vi "Vision Processing.vi"(4 "error in (no error)":errorcluster, 6 "CameraDevRef":T1) -> ()   [LabVIEW 2011]
uses:
  <vilib>/Rock Robotics/WPI/Camera/WPI_CameraDevRef.ctl
  Robot Global Data.vi
  <vilib>/vision/NI_Vision_Development_Module.lvlib
panel:
  in  "Run Calculations":bool
  in  "Manual Overide":bool
  out "Raw Turret":dbl
  out "Target X Coord":dbl
  out "Target Distance":dbl
  out "Target Y Coord":dbl
  out "Distance Array":dbl[](array[numeric])
  in  "Scaler":dbl=0.85
  in  "Lower Speed Limit":dbl=0.05
  out "Number of Rectangles Visible":dbl
  out "Y Position Array":dbl[](array[numeric])
  out "X Position Array":dbl[](array[numeric])
  in  "View":bool
  out "Target Info":T2(array[cluster])
  in  "Area Size Limit":i32=444
  in  "Particle Count Limit":i32=8
  in  "Score Limits":T3={"Rect Coverage"=76.0, "Aspect Ratio"=40.0, "X Edge Strength"=40.0, "Y Edge Strength"=60.0}
  in  "Processing":enum32{"Color", "Intensity", "Intensity Open"}(tab)=enum."Intensity Open"
  in  "Luminance":i32=255
  in  "Saturation":i32=255
  in  "Hue":i32(knob)=65 scale=0.0..255.0
  in  "Margins":cluster{"Hue":i32, "Sat":i32, "Lum":i32}={"Hue"=20, "Sat"=27, "Lum"=30} {"Sat" scale=0.0..40.0; "Lum" scale=0.0..40.0; "Hue" scale=0.0..40.0}
  in  "Range":cluster{"Lower value":sgl, "Upper value":sgl}={"Lower value"=150.0, "Upper value"=255.0} {"Lower value" scale=0.0..255.0; "Upper value" scale=0.0..255.0}
  in  "Range":cluster{"Lower value":sgl, "Upper value":sgl}={"Lower value"=123.804344, "Upper value"=255.0} {"Lower value" scale=0.0..255.0; "Upper value" scale=0.0..255.0}
  in  "View":bool
  out "Processed Image":T4(plugin-control)
  out "Original Image":T4(plugin-control)
  # "Instructions:\nProcessing the reflective tape that is illuminated by a ring light can be based\non color or light intensity.\nParticles within the image are scored by rectangle coverage, aspect ratio, and\nfor being hollow with a bold edge. A particle is considered a target if all scores\nare above the score limits. Particles can be annotated -- surrounded by\na rectangle and scores drawn to the left .\nTo control the number of particles being scored, use the count limit and the size\nlimit."
  # "To debug, Enable using the View button.\nFor color processing, you can click in the image to select the color for processing."
  # "Enable by clicking the View button.\nGreen scores are above the limit, orange are below. Inner/outer rect\nindicates all passed."
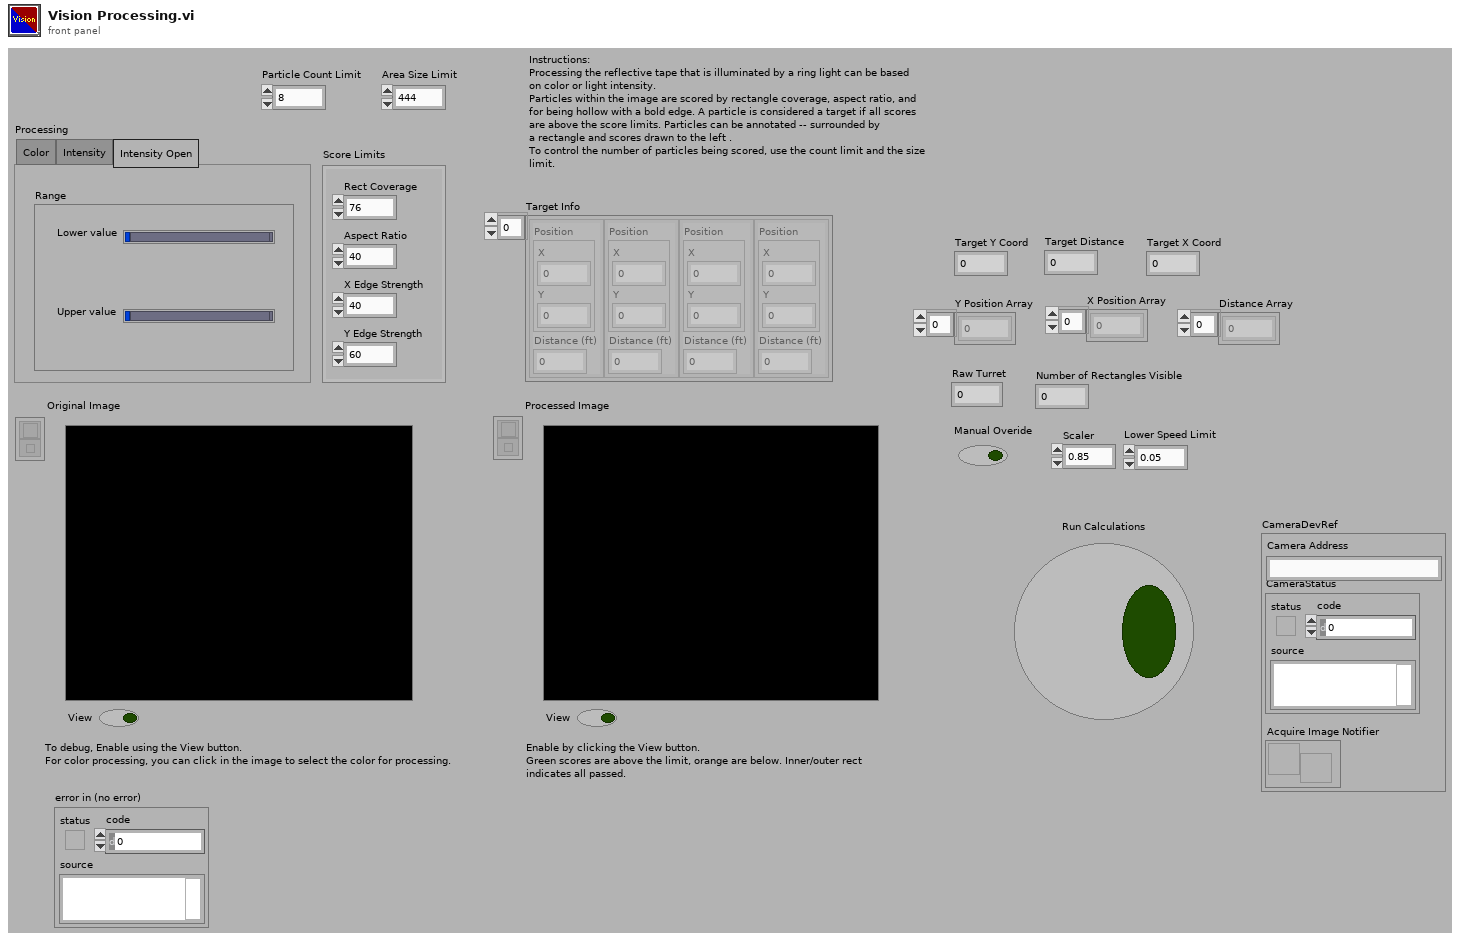
[diagram p1: front panel]
types:
  T1 = typedef "WPI_CameraDevRef.ctl" = cluster{"Camera Address":string, "CameraStatus":errorcluster, "Acquire Image Notifier":refnum<notifier>}
  T2 = cluster{"Position":cluster{"X":dbl, "Y":dbl}, "Distance (ft)":dbl}[]
  T3 = cluster{"Rect Coverage":dbl, "Aspect Ratio":dbl, "X Edge Strength":dbl, "Y Edge Strength":dbl}
  T4 = typedef "IMAQ Image.ctl" = refnum<image>
  T5 = typedef "Image Type" = u32
  T6 = enum32{"AutoM", "Close", "Dilate", "Erode", "Gradient", "Gradient out", "Gradient in", "Hit miss", "Open", "PClose", "POpen", "Thick", "Thin"}
  T7 = typedef "WPI_CameraImageSize.ctl" = enum16{"640x480", "320x240", "160x120"}
  T8 = cluster{"fps":i32, "compression":i32, "Image Size":T7}
  T9 = cluster{cluster{"Left":dbl, "Top":dbl, "Right":dbl, "Bottom":dbl}, dbl[]}[]
  T10 = cluster{"Left":dbl, "Top":dbl, "Right":dbl, "Bottom":dbl}
  T11 = cluster{"Target Center (-1 to 1)":cluster{"X":dbl, "Y":dbl}, "Distance (ft)":dbl}
  T12 = cluster{"Target Center (-1 to 1)":cluster{"X":dbl, "Y":dbl}, "Distance (ft)":dbl}[]
  T13 = cluster{"Axis 1":dbl, "Axis 2":dbl, "Axis 3":dbl, "Axis 4":dbl, "Axis 5":dbl, "Axis 6":dbl, "Button 1":bool, "Button 2":bool, "Button 3":bool, "Button 4":bool, "Button 5":bool, "Button 6":bool, "Button 7":bool, "Button 8":bool, "Button 9":bool, "Button 10":bool, "Button 11":bool, "Button 12":bool}
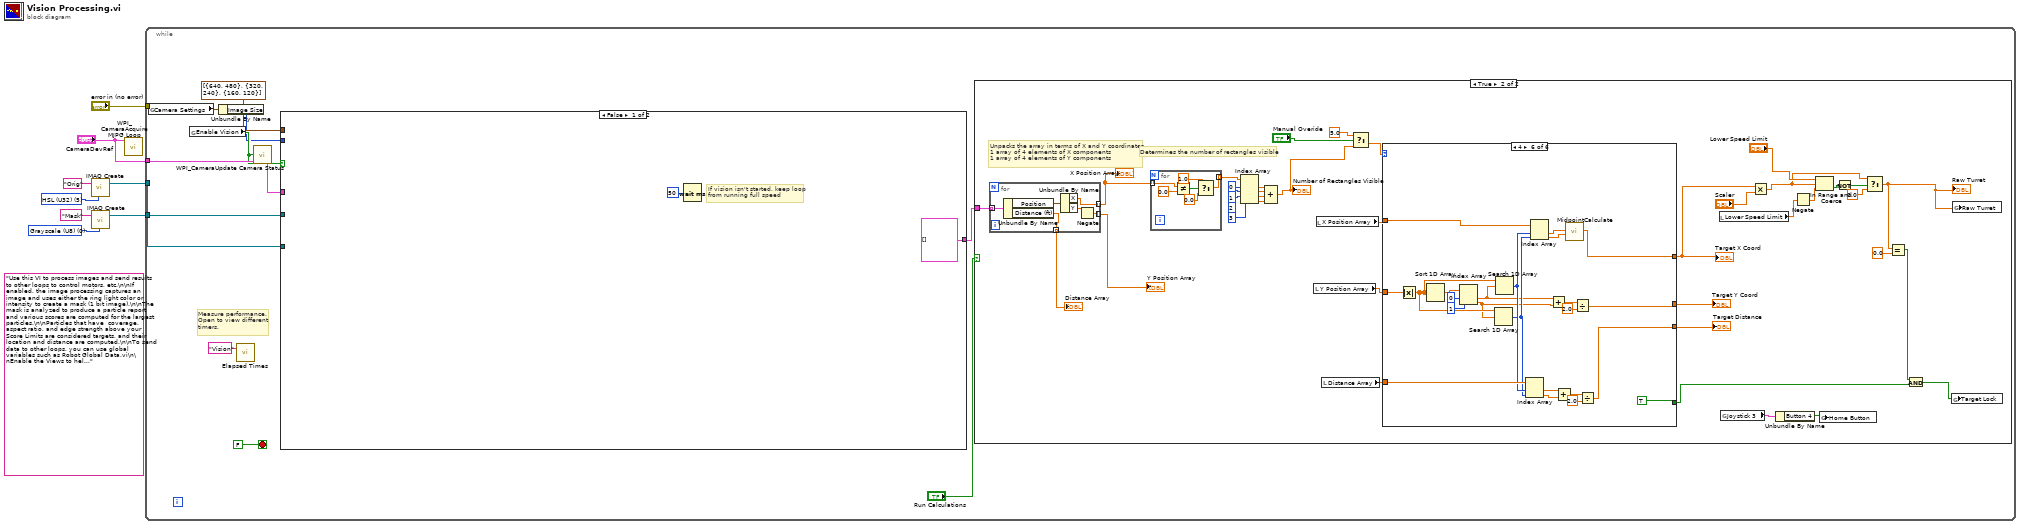
[diagram p0: block diagram]
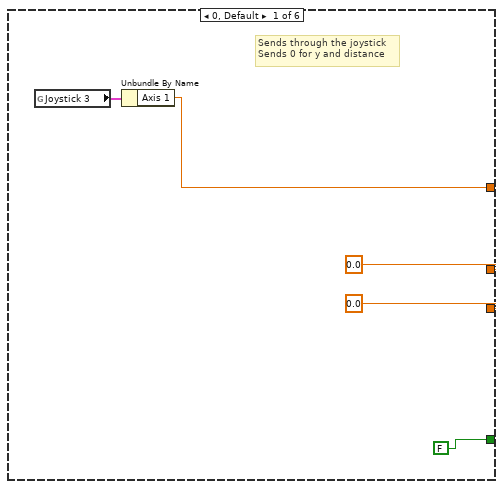
[diagram p3: hidden frame]
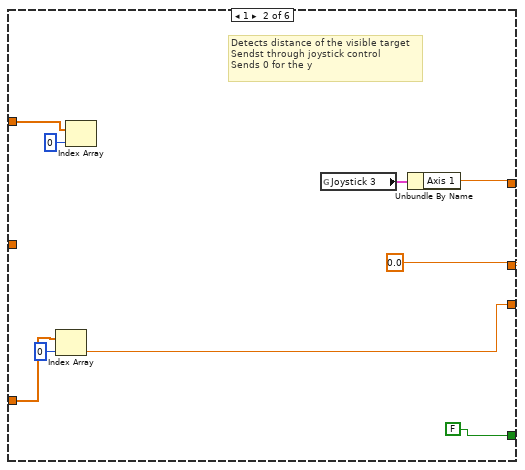
[diagram p4: hidden frame]
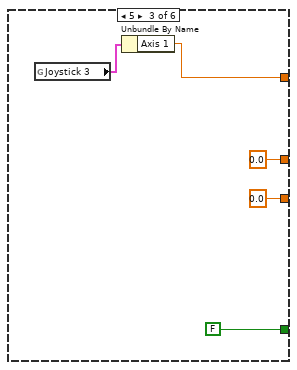
[diagram p5: hidden frame]
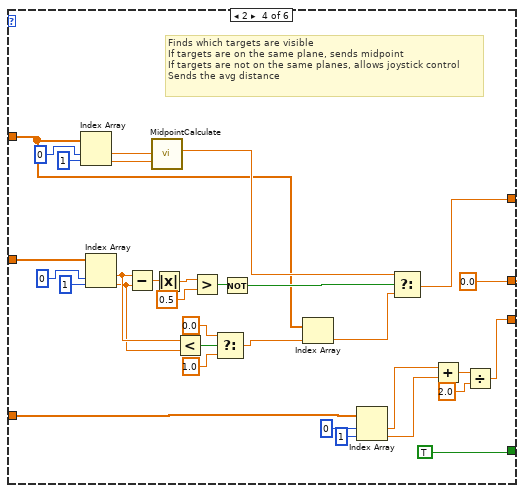
[diagram p6: hidden frame]
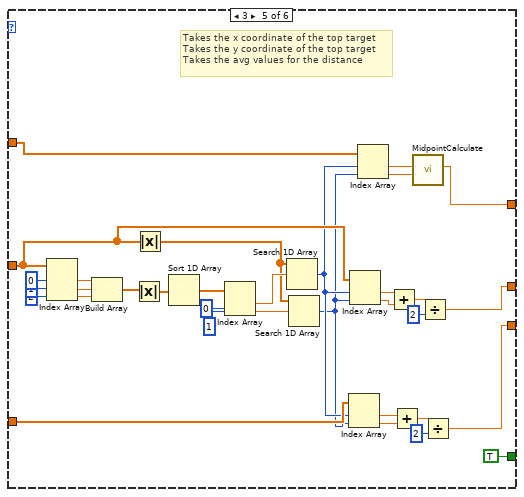
[diagram p7: hidden frame]
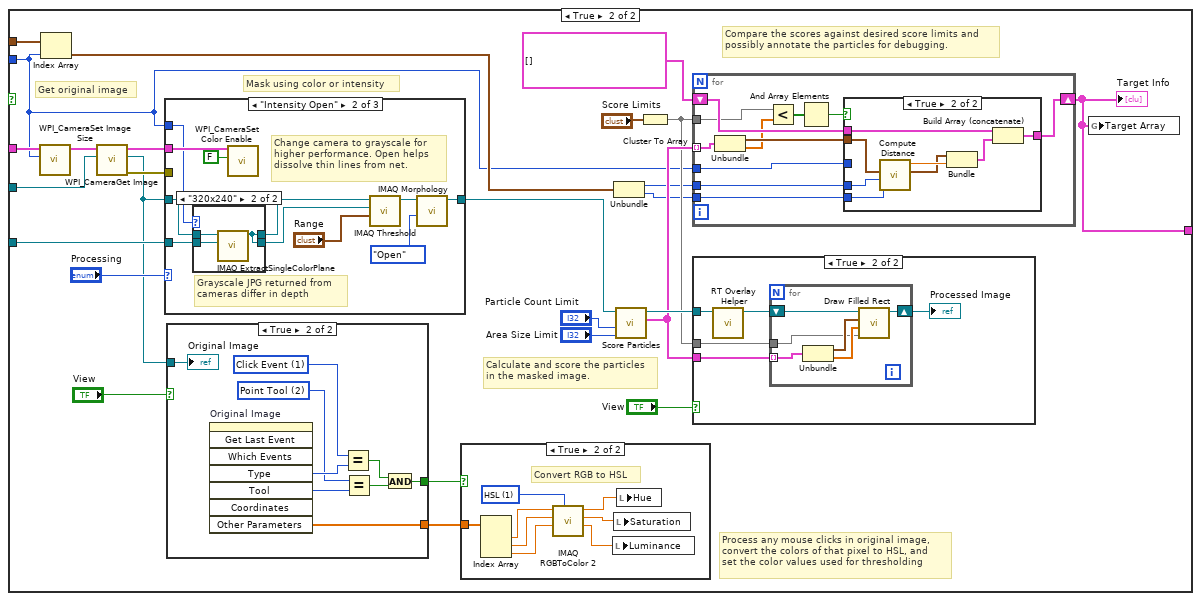
[diagram p8: hidden frame]
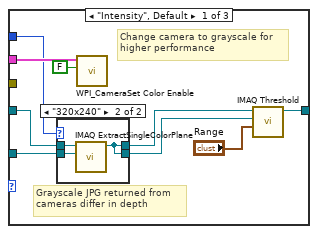
[diagram p10: hidden frame]
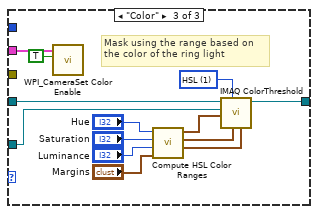
[diagram p13: hidden frame]
diagram:
  w3 = T5 0 items=["Grayscale (U8)", "Grayscale (I16)", "Grayscale (SGL)", "Complex (CSG)", "RGB (U32)", "HSL (U32)", "RGB (U64)", "Grayscale (U16)"] ("Image Type")
  (unwired) "Use this VI to process images and send results to other loops to control motors, etc.\n\nIf enabled, the image processing captures an image and uses either the ring light color or intensity to create a mask (1 bit image).\n\nThe mask is analyzed to produce a particle report and various scores are computed for the largest particles.\n\nParticles that have  coverage, aspect ratio, and edge strength above your Score Limits are considered targets, and their location and distance are computed.\n\nTo send data to other loops, you can use global variables such as Robot Global Data.vi\n\nEnable the Views to help debug color settings. Disable the View to speed up processing."
  w7 = T5 5 items=["Grayscale (U8)", "Grayscale (I16)", "Grayscale (SGL)", "Complex (CSG)", "RGB (U32)", "HSL (U32)", "RGB (U64)", "Grayscale (U16)"] ("Image Type")
  n1 = call "IMAQ Create"("Image Name"="Orig", "Image Type"=w7) -> ("New Image"=w6:T4)  [unwired: 2 in, 2 out]
  n2 = call "IMAQ Create"("Image Name"="Mask", "Image Type"=w3) -> ("New Image"=w1:T4)  [unwired: 2 in, 2 out]
  n3 = call <vilib>:"WPI_CameraAcquire MJPG Loop.vi"("CameraDevRef"="CameraDevRef") -> ()  [unwired: 11 in]
  n4 = while {
    tunnel: w6 -> [w19]
    tunnel: "CameraDevRef" -> [w18]
    tunnel: "error in (no error)" -> [_]
    tunnel: w1 -> [w14]
    stop <- FALSE stop-if-true
    # "Measure performance.\nOpen to view different\ntimers."
    n5 = global read "Robot Global Data.vi" "Camera Settings"() -> (w12:T8)
    n6 = global read "Robot Global Data.vi" "Enable Vision"() -> (w16:bool)
    n7 = Unbundle By Name(w12) -> ("Image Size"=w11:T7)
    n8 = call "Elapsed Times.vi"("Call Name"="Vision") -> ()  [unwired: 2 in, 1 out]
    n9 = call <vilib>:"WPI_CameraUpdate Camera Status.vi"("CameraDevRef In"=w18, "Enable Vision"=w16) -> ("CameraDevRef Out"=w17:T1)  [unwired: 3 in]
    n10 = case shown="False" w16 {
      tunnel: w19 -> [_ w196]
      tunnel: w17 -> [_ w192]
      tunnel: w14 -> [_ w183]
      tunnel: cluster{i32, i32}[] [{640, 480}, {320, 240}, {160, 120}] -> [_ w187]
      tunnel: w11 -> [_ w180]
      tunnel: [T2 [] w181] -> w10
      frame False {
        # "If vision isn't started, keep loop\nfrom running full speed"
        n11 = Wait (ms)(milliseconds to wait=u32 50) -> ()  [unwired: 1 out]
      }
      frame True {
        # "Compare the scores against desired score limits and\npossibly annotate the particles for debugging."
        # "Process any mouse clicks in original image,\nconvert the colors of that pixel to HSL, and\nset the color values used for thresholding"
        # "Calculate and score the particles\nin the masked image."
        # "Mask using color or intensity"
        # "Get original image"
        n12 = call <vilib>:"WPI_CameraSet Image Size.vi"("Image Size"=w180, "CameraDevRef"=w192) -> ("CameraDevRef Out"=w193:T1)  [unwired: 8 in, 1 out]
        n13 = Index Array(array=w187, index=w180) -> (element=w184:cluster{i32, i32})
        n14 = call <vilib>:"WPI_CameraGet Image.vi"("Image"=w196, "CameraDevRef"=w193) -> ("error out"=w194:errorcluster, "Image Out"=w182:T4, "CameraDevRef Out"=w195:T1)  [unwired: 7 in]
        n15 = case shown="\"Intensity Open\"" "Processing" {
          tunnel: w182 -> [w218 w230 w256]
          tunnel: [w221 w235 w255] -> w190
          tunnel: w195 -> [w219 w233 w246]
          tunnel: w194 -> [_ _ _]
          tunnel: w183 -> [w217 w231 w244]
          tunnel: w180 -> [w216 w232 _]
          frame "Intensity", Default {
            # "Grayscale JPG returned from\ncameras differ in depth"
            # "Change camera to grayscale for\nhigher performance"
            n16 = case shown="\"320x240\"" w216 {
              tunnel: w218 -> [w224 w227]
              tunnel: w217 -> [w223 w226]
              tunnel: [w224 w225] -> w215
              tunnel: [w223 w225] -> w214
              frame "640x480", Default {
              }
              frame "320x240" {
                n17 = call "IMAQ ExtractSingleColorPlane"("Image Dst"=w226, "Image Src"=w227) -> ("Image Dst Out"=w225:T4)  [unwired: 8 in, 1 out]
              }
            }
            n18 = call <vilib>:"WPI_CameraSet Color Enable.vi"("Color Enabled"=FALSE, "CameraDevRef"=w219) -> ()  [unwired: 8 in, 2 out]
            n19 = call "IMAQ Threshold"("Range"="Range", "Image Dst"=w214, "Image Src"=w215) -> ("Image Dst Out"=w221:T4)  [unwired: 3 in, 5 out]
          }
          frame "Intensity Open" {
            # "Grayscale JPG returned from\ncameras differ in depth"
            # "Change camera to grayscale for\nhigher performance. Open helps\ndissolve thin lines from net."
            n20 = case shown="\"320x240\"" w232 {
              tunnel: w230 -> [w240 w243]
              tunnel: w231 -> [w239 w242]
              tunnel: [w240 w241] -> w229
              tunnel: [w239 w241] -> w228
              frame "640x480", Default {
              }
              frame "320x240" {
                n21 = call "IMAQ ExtractSingleColorPlane"("Image Dst"=w242, "Image Src"=w243) -> ("Image Dst Out"=w241:T4)  [unwired: 8 in, 1 out]
              }
            }
            n22 = call <vilib>:"WPI_CameraSet Color Enable.vi"("Color Enabled"=FALSE, "CameraDevRef"=w233) -> ()  [unwired: 8 in, 2 out]
            n23 = call "IMAQ Threshold"("Range"="Range", "Image Dst"=w228, "Image Src"=w229) -> ("Image Dst Out"=w236:T4)  [unwired: 3 in, 5 out]
            n24 = call "IMAQ Morphology"("Operation"=T6."Open", "Image Src"=w236) -> ("Image Dst Out"=w235:T4)  [unwired: 8 in, 1 out]
          }
          frame "Color" {
            w254 = u16 1 items=["RGB", "HSL", "HSV", "HSI"] ("Color Mode")
            # "Mask using the range based on\nthe color of the ring light"
            n25 = call <vilib>:"WPI_CameraSet Color Enable.vi"("Color Enabled"=TRUE, "CameraDevRef"=w246) -> ()  [unwired: 8 in, 2 out]
            n26 = call "Compute HSL Color Ranges.vi"("Margins"="Margins", "Luminance"="Luminance", "Saturation"="Saturation", "Hue"="Hue") -> ("Lum Range"=w251:cluster{i32, i32}, "Sat Range"=w252:cluster{i32, i32}, "Hue Range"=w253:cluster{i32, i32})  [unwired: 5 in]
            n27 = call "IMAQ ColorThreshold"("Blue or Luma or Val or Inten Range"=w251, "Green or Sat Range"=w252, "Color Mode"=w254, "Red or Hue Range"=w253, "Image Dst"=w244, "Image Src"=w256) -> ("Image Dst Out"=w255:T4)  [unwired: 4 in, 1 out]
          }
        }
        n28 = case shown="True" "View" {
          tunnel: w182 -> [_ w276]
          tunnel: [_ w271] -> w189
          tunnel: [_ w268] -> w188
          frame False {
          }
          frame True {
            w269 = 2 items=["None", "Selection Tool", "Point Tool", "Line Tool", "Rectangle Tool", "Oval Tool", "Polygon Tool", "ClosedFreehandTool", "Annulus Tool", "Rotated Rectangle Tool", "Zoom Tool", "Pan Tool", "Polyline Tool", "Freehand Tool"] ("Tool")
            w270 = 1 items=["No Event"=0, "Click Event"=1, "Draw Event"=2, "Size Event"=4, "Scroll Event"=5, "Double Click Event"=8] ("Type")
            n29 = invoke on="Original Image" class="ImageControl" method="Get Last Event"() -> ("Type"=w272:i32, "Tool"=w275:i32, "Other Parameters"=w268:sgl[])  [unwired: 8 in, 5 out]
            n30 = Equal?(x=w270, y=w272) -> (x = y?=w273:bool)
            n31 = Equal?(x=w269, y=w275) -> (x = y?=w274:bool)
            n32 = And(x=w273, y=w274) -> (x .and. y?=w271:bool)
            "Original Image" <- w276
          }
        }
        n33 = case shown="True" w189 {
          tunnel: w188 -> [_ w213]
          frame False {
          }
          frame True {
            w212 = u16 1 items=["RGB", "HSL", "HSV", "HSI", "CIE L*a*b*", "CIE XYZ"] ("Color Mode")
            # "Convert RGB to HSL"
            n34 = Index Array(array=w213) -> (element #1=w211:sgl, element #2=w209:sgl, element #3=w207:sgl)  [unwired: 3 in]
            n35 = call "IMAQ RGBToColor 2"("Color Mode"=w212, "Blue value"=w207, "Green value"=w209, "Red value"=w211) -> ("Blue or Luma or Val or Inten or Z or b*value"=w206:dbl, "Green or Sat or Y or a* value"=w208:dbl, "Red or Hue or X or L* value"=w210:dbl)  [unwired: 4 in, 1 out]
            n36 = local write "Luminance"(w206) -> ()
            n37 = local write "Saturation"(w208) -> ()
            n38 = local write "Hue"(w210) -> ()
          }
        }
        n39 = Unbundle(w184) -> (w186:i32, w185:i32)
        n40 = call "Score Particles.vi"("Area Size Limit"="Area Size Limit", "Particle Count Limit"="Particle Count Limit", "Image Refnum in"=w190) -> ("Scored Particle Info"=w201:T9, "Image Refnum out"=w204:T4)  [unwired: 7 in]
        n41 = Cluster To Array(cluster="Score Limits") -> (array=w199:dbl[])
        n42 = for {
          shift-right: [w286] -> w181
          shift-left: T2 [] -> [w287]
          tunnel: w186 -> [w285]
          tunnel: w201 -> [w283] mode=indexing
          tunnel: w199 -> [w278]
          tunnel: w180 -> [w282]
          tunnel: w185 -> [w277]
          n43 = Unbundle(w283) -> (w284:T10, w279:dbl[])
          n44 = Less?(x=w278, y=w279) -> (x < y?=w281:bool[])
          n45 = And Array Elements(Boolean array=w281) -> (logical AND=w280:bool)
          n46 = case shown="True" w280 {
            tunnel: w287 -> [w288 w296]
            tunnel: [w288 w295] -> w286
            tunnel: w284 -> [_ w291]
            tunnel: w285 -> [_ w293]
            tunnel: w282 -> [_ _]
            tunnel: w277 -> [_ w290]
            frame False {
            }
            frame True {
              n47 = call "Compute Distance.vi"("Y Image Resolution"=w290, "X Image Resolution"=w293, "Bounding Box"=w291) -> ("Target Center (-1 to 1)"=w289:cluster{"X":dbl, "Y":dbl}, "Distance (ft)"=w292:dbl)  [unwired: 7 in]
              n48 = Bundle("Target Center (-1 to 1)"=w289, "Distance (ft)"=w292) -> (w294:T11)  [unwired: 1 in]
              n49 = Build Array (concatenate)(w296, w294) -> (w295:T12)
            }
          }
        }
        "Target Info" <- w181
        n50 = case shown="True" "View" {
          tunnel: w204 -> [_ w258]
          tunnel: w201 -> [_ w260]
          tunnel: w199 -> [_ w259]
          frame False {
          }
          frame True {
            n51 = call "RT Overlay Helper.vi"("Refnum in"=w258) -> ("Refnum out"=w261:T4)  [unwired: 10 in]
            n52 = for {
              shift-right: [w266] -> w257
              shift-left: w261 -> [w267]
              tunnel: w260 -> [w263] mode=indexing
              tunnel: w259 -> [w262]
              n53 = Unbundle(w263) -> (w264:T10, w265:dbl[])
              n54 = call "Draw Filled Rect.vi"("Limits"=w262, "Scores"=w265, "Bounding Box"=w264, "image in"=w267) -> ("image out"=w266:T4)  [unwired: 7 in]
            }
            "Processed Image" <- w257
          }
        }
        n55 = global write "Robot Global Data.vi" "Target Array"(w181) -> ()
      }
    }
    n56 = case shown="True" "Run Calculations" {
      tunnel: w10 -> [_ w29]
      frame False {
      }
      frame True {
        # "Determines the number of rectangles visible"
        # "Unpacks the array in terms of X and Y coordinates\n1 array of 4 elements of X components\n1 array of 4 elements of Y components"
        n57 = for {
          tunnel: [w175] -> w30 mode=indexing
          tunnel: [w176] -> w40 mode=indexing
          tunnel: w29 -> [w173] mode=indexing
          tunnel: [w172] -> w49 mode=indexing
          n58 = Unbundle By Name(w173) -> ("Position"=w177:cluster{"X":dbl, "Y":dbl}, "Distance (ft)"=w172:dbl)
          n59 = Unbundle By Name(w177) -> ("X"=w176:dbl, "Y"=w174:dbl)
          n60 = Negate(x=w174) -> (-x=w175:dbl)
        }
        "X Position Array" <- w40
        "Y Position Array" <- w30
        "Distance Array" <- w49
        n61 = for {
          tunnel: w40 -> [w63] mode=indexing
          tunnel: [w59] -> w39 mode=indexing
          n62 = Not Equal?(x=w63, y=0.0) -> (x != y?=w62:bool)
          n63 = Select(t=1.0, s=w62, f=0.0) -> (s? t:f=w59:dbl)
        }
        n64 = Index Array(array=w39, index #1=0 ("index"), index #2=1 ("index"), index #3=2 ("index"), index #4=3 ("index")) -> (element #1=w37:dbl, element #2=w38:dbl, element #3=w36:dbl, element #4=w35:dbl)
        n65 = Compound Arithmetic op=ADD(w37, w38, w36, w35) -> (w28:dbl)
        "Number of Rectangles Visible" <- w28
        n66 = local read "Y Position Array"() -> (w53:dbl[])
        n67 = local read "X Position Array"() -> (w41:dbl[])
        n68 = local read "Distance Array"() -> (w54:dbl[])
        n69 = Select(t=5.0, s="Manual Overide", f=w28) -> (s? t:f=w57:dbl)
        n70 = case shown="4" w57 {
          tunnel: w41 -> [_ w73 _ w86 w132 w165]
          tunnel: [w68 w71 w82 w104 w129 w155] -> w52
          tunnel: [0.0 ("X") 0.0 ("X") 0.0 ("X") 0.0 ("X") w133 w154] -> w50
          tunnel: [0.0 ("X") w76 0.0 ("X") w97 w117 w149] -> w51
          tunnel: w53 -> [_ _ _ w113 w125 w170]
          tunnel: w54 -> [_ w78 _ w96 w120 w164]
          tunnel: [FALSE FALSE FALSE TRUE TRUE TRUE] -> w25
          frame 0, Default {
            # "Sends through the joystick\nSends 0 for y and distance"
            n71 = global read "Robot Global Data.vi" "Joystick 3"() -> (w69:T13)
            n72 = Unbundle By Name(w69) -> ("Axis 1"=w68:dbl)
          }
          frame 1 {
            # "Detects distance of the visible target\nSendst through joystick control\nSends 0 for the y"
            n73 = Index Array(array=w78, index=0) -> (element=w76:dbl)
            n74 = Index Array(array=w73, index=0) -> ()  [unwired: 1 out]
            n75 = global read "Robot Global Data.vi" "Joystick 3"() -> (w72:T13)
            n76 = Unbundle By Name(w72) -> ("Axis 1"=w71:dbl)
          }
          frame 5 {
            n77 = global read "Robot Global Data.vi" "Joystick 3"() -> (w83:T13)
            n78 = Unbundle By Name(w83) -> ("Axis 1"=w82:dbl)
          }
          frame 2 {
            # "Finds which targets are visible\nIf targets are on the same plane, sends midpoint\nIf targets are not on the same planes, allows joystick control\nSends the avg distance"
            n79 = Index Array(array=w86, index #1=0 ("index"), index #2=1 ("index")) -> (element #1=w102:dbl, element #2=w101:dbl)
            n80 = Index Array(array=w113, index #1=0 ("index"), index #2=1 ("index")) -> (element #1=w92:dbl, element #2=w91:dbl)
            n81 = Subtract(x=w92, y=w91) -> (x-y=w110:dbl)
            n82 = call "MidpointCalculate.vi"("X2"=w101, "X1"=w102) -> ("Midpoint"=w105:dbl)  [unwired: 9 in]
            n83 = Absolute Value(x=w110) -> (abs(x)=w109:dbl)
            n84 = Less?(x=w92, y=w91) -> (x < y?=w90:bool)
            n85 = Greater?(x=w109, y=0.5) -> (0:w106:bool)
            n86 = Select(t=0.0, s=w90, f=1.0) -> (s? t:f=w87:dbl)
            n87 = Not(x=w106) -> (.not. x?=w107:bool)
            n88 = Index Array(array=w86, index=w87) -> (element=w85:dbl)
            n89 = Index Array(array=w96, index #1=0 ("index"), index #2=1 ("index")) -> (element #1=w95:dbl, element #2=w94:dbl)
            n90 = Select(t=w105, s=w107, f=w85) -> (s? t:f=w104:dbl)
            n91 = Add(x=w95, y=w94) -> (x+y=w100:dbl)
            n92 = Divide(x=w100, y=2.0) -> (x/y=w97:dbl)
          }
          frame 3 {
            # "Takes the x coordinate of the top target\nTakes the y coordinate of the top target\nTakes the avg values for the distance"
            n93 = Index Array(array=w125, index #1=0 ("index"), index #2=1 ("index"), index #3=2 ("index")) -> (element #1=w145:dbl, element #2=w144:dbl, element #3=w143:dbl)
            n94 = Build Array(w145, w144, w143) -> (w142:dbl[])
            n95 = Absolute Value(x=w142) -> (abs(x)=w136:dbl[])
            n96 = Absolute Value(x=w125) -> (abs(x)=w128:dbl[])
            n97 = Sort 1D Array(array=w136) -> (sorted array=w141:dbl[])
            n98 = Index Array(array=w141, index #1=0 ("index"), index #2=1 ("index")) -> (element #1=w137:dbl, element #2=w138:dbl)
            n99 = Search 1D Array(1D array=w128, element=w137) -> (index of element=w119:i32)  [unwired: 1 in]
            n100 = Search 1D Array(1D array=w128, element=w138) -> (index of element=w118:i32)  [unwired: 1 in]
            n101 = Index Array(array=w120, index #1=w119, index #2=w118) -> (element #1=w122:dbl, element #2=w121:dbl)
            n102 = Index Array(array=w125, index #1=w119, index #2=w118) -> (element #1=w127:dbl, element #2=w126:dbl)
            n103 = Index Array(array=w132, index #1=w119, index #2=w118) -> (element #1=w131:dbl, element #2=w130:dbl)
            n104 = Add(x=w127, y=w126) -> (x+y=w135:dbl)
            n105 = Add(x=w122, y=w121) -> (x+y=w123:dbl)
            n106 = call "MidpointCalculate.vi"("X2"=w130, "X1"=w131) -> ("Midpoint"=w129:dbl)  [unwired: 9 in]
            n107 = Divide(x=w135, y=2) -> (x/y=w133:dbl)
            n108 = Divide(x=w123, y=2) -> (x/y=w117:dbl)
          }
          frame 4 {
            n109 = Absolute Value(x=w170) -> (abs(x)=w166:dbl[])
            n110 = Sort 1D Array(array=w166) -> (sorted array=w169:dbl[])
            n111 = Index Array(array=w169, index #1=0 ("index"), index #2=1 ("index")) -> (element #1=w161:dbl, element #2=w160:dbl)
            n112 = Search 1D Array(1D array=w166, element=w160) -> (index of element=w162:i32)  [unwired: 1 in]
            n113 = Search 1D Array(1D array=w166, element=w161) -> (index of element=w163:i32)  [unwired: 1 in]
            n114 = Index Array(array=w164, index #1=w163, index #2=w162) -> (element #1=w151:dbl, element #2=w150:dbl)
            n115 = Index Array(array=w165, index #1=w163, index #2=w162) -> (element #1=w157:dbl, element #2=w156:dbl)
            n116 = Add(x=w161, y=w160) -> (x+y=w159:dbl)
            n117 = Add(x=w151, y=w150) -> (x+y=w152:dbl)
            n118 = call "MidpointCalculate.vi"("X2"=w156, "X1"=w157) -> ("Midpoint"=w155:dbl)  [unwired: 9 in]
            n119 = Divide(x=w159, y=2.0) -> (x/y=w154:dbl)
            n120 = Divide(x=w152, y=2.0) -> (x/y=w149:dbl)
          }
        }
        "Target Y Coord" <- w50
        "Target Distance" <- w51
        "Target X Coord" <- w52
        n121 = local read "Lower Speed Limit"() -> (w43:dbl)
        n122 = global read "Robot Global Data.vi" "Joystick 3"() -> (w22:T13)
        n123 = Multiply(x=w52, y="Scaler") -> (x*y=w48:dbl)
        n124 = Unbundle By Name(w22) -> ("Button 4"=w21:bool)
        n125 = Negate(x=w43) -> (-x=w44:dbl)
        n126 = In Range and Coerce(upper limit="Lower Speed Limit", x=w48, lower limit=w44) -> (In Range?=w45:bool)  [unwired: 1 out]
        n127 = global write "Robot Global Data.vi" "Home Button"(w21) -> ()
        n128 = Not(x=w45) -> (.not. x?=w46:bool)
        n129 = Select(t=w48, s=w46, f=0.0) -> (s? t:f=w27:dbl)
        "Raw Turret" <- w27
        n130 = Equal?(x=w27, y=0.0) -> (x = y?=w24:bool)
        n131 = And(x=w24, y=w25) -> (x .and. y?=w23:bool)
        n132 = global write "Robot Global Data.vi" "Target Lock"(w23) -> ()
        n133 = global write "Robot Global Data.vi" "Raw Turret"(w27) -> ()
      }
    }
  }
